vi "Retrieve from FIFO.vi"(8 "error in (no error)":errorcluster, 9 "timeout in ms (0)":i32 format="%d ms", 10 "expected iteration":u64, 11 "Transfer Group in":refnum<class "Transfer Group.lvclass">) -> (0 "error out":errorcluster, 1 "late":bool, 2 "ready":bool, 3 "Transfer Group out":refnum<class "Transfer Group.lvclass">)   [LabVIEW 2017, in "DSF Core.lvlib" / "Transfer Group.lvclass"]
uses:
  Transfer Group.lvclass
  Invalid Iteration Error.vi
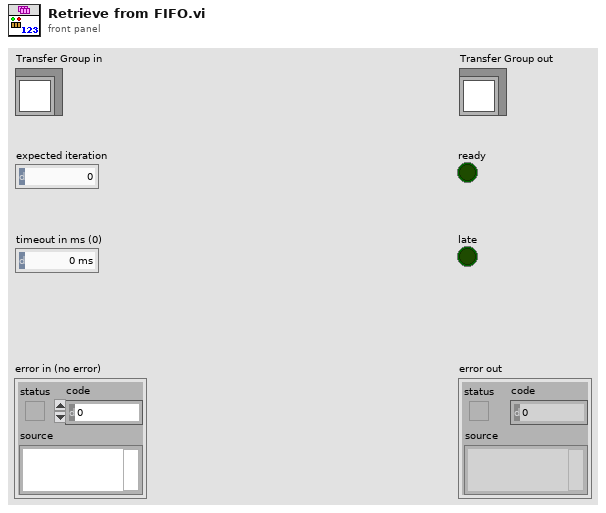
[diagram p1: front panel]
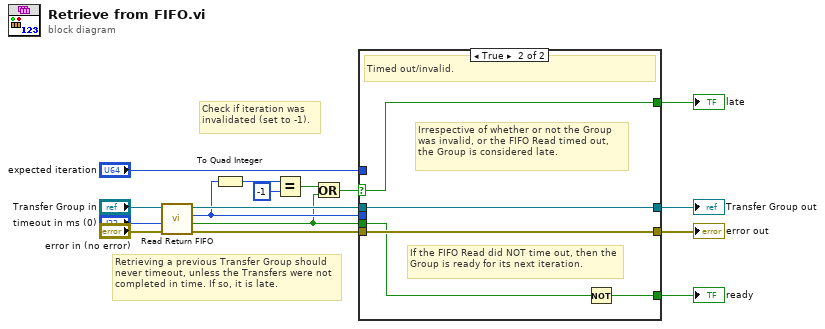
[diagram p0: block diagram]
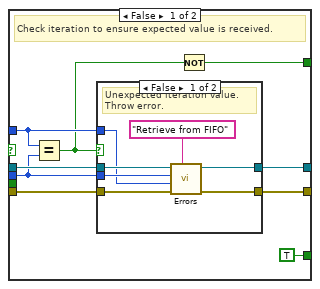
[diagram p2: hidden frame]
diagram:
  # "Check if iteration was invalidated (set to -1)."
  # "Retrieving a previous Transfer Group should never timeout, unless the Transfers were not completed in time. If so, it is late."
  n1 = call "Read Return FIFO.vi"("error in (no error)"="error in (no error)", "timeout in ms (0)"="timeout in ms (0)", "Transfer Group in"="Transfer Group in") -> ("error out"=w16:errorcluster, "timed out?"=w1:bool, "Transfer Group iteration"=w4:u64, "Transfer Group out"=w8:refnum<class "Transfer Group.lvclass">)  [unwired: 5 in]
  n2 = To Quad Integer(1:w4) -> (0:w6:i64)
  n3 = Equal?(x=w6, y=i64 -1) -> (x = y?=w3:bool)
  n4 = Or(x=w3, y=w1) -> (x .or. y?=w2:bool)
  n5 = case shown="True" w2 {
    selector: w2 -> [_ w35]
    tunnel: w16 -> [w23 w39]
    tunnel: w8 -> [w25 w38]
    tunnel: w4 -> [w21 _]
    tunnel: "expected iteration" -> [w20 _]
    tunnel: [w22 w39] -> w10
    tunnel: [w24 w38] -> w9
    tunnel: [TRUE w37] -> w12
    tunnel: [w19 w35] -> w7
    tunnel: w1 -> [_ w36]
    frame False {
      # "Check iteration to ensure expected value is received."
      n6 = Equal?(x=w20, y=w21) -> (x = y?=w18:bool)
      n7 = case shown="False" w18 {
        tunnel: w25 -> [w32 w33]
        tunnel: [w30 w33] -> w24
        tunnel: w23 -> [w31 w34]
        tunnel: [w29 w34] -> w22
        tunnel: w21 -> [w28 _]
        tunnel: w20 -> [w27 _]
        frame False {
          # "Unexpected iteration value. Throw error."
          n8 = call-poly "Errors.vi"("error source vi name"="Retrieve from FIFO", "error in (no error)"=w31, "expected iteration"=w27, "actual iteration"=w28, "Transfer Group in"=w32) -> ("error out"=w29:errorcluster, "Transfer Group out"=w30:refnum<class "Transfer Group.lvclass">)  [unwired: 5 in]
        }
        frame True {
          # "Expected value. Proceed."
        }
      }
      n9 = Not(x=w18) -> (.not. x?=w19:bool)
    }
    frame True {
      # "Irrespective of whether or not the Group was invalid, or the FIFO Read timed out, the Group is considered late."
      # "If the FIFO Read did NOT time out, then the Group is ready for its next iteration."
      # "Timed out/invalid."
      n10 = Not(x=w36) -> (.not. x?=w37:bool)
    }
  }
  "error out" <- w10
  "Transfer Group out" <- w9
  "ready" <- w12
  "late" <- w7
